vi "DIBPowerCheck_t.vi"(0 "TSM context":T2, 5 "DIBPowerCheck_TC":T1={"Voltage Limit, V"=24.0, "Current Level (A)"=0.05}) -> (15 "error out":errorcluster)   [LabVIEW 2019]
uses:
  <vilib>/NI_TestStand_SemiconductorModule/NI_TestStand_Semiconductor_Module.lvlibp/PinMap/General/SemiconductorModuleContext.ctl
  typedefs/DIBPowerCheck_TC.ctl
  typedefs/DIBPowerCheck_PC.ctl
  Common/Instrument Control/DCPower/TSM/TSM SSC DCPower.ctl
  <vilib>/NI_TestStand_SemiconductorModule/NI_TestStand_Semiconductor_Module.lvlibp/PinMap/PinQueryContext/MultiplePinMultipleSessionQueryContext/MultiplePinMultipleSessionQueryContext.lvclass
  C:/Program Files/National Instruments/LabVIEW 2019/vi.lib/NI_TestStand_SemiconductorModule/NI_TestStand_Semiconductor_Module.lvlibp/PinMap/PinQueryContext/PinQueryContext.lvclass
  Common/Instrument Control/DCPower/SSC DCPower/SSC DCPower.ctl
  Common/Instrument Control/Shared SubVIs/TSM Pin Abstraction/TSM Pin Information.ctl
  Common/Instrument Control/Shared SubVIs/TSM Pin Abstraction/TSM Pin Type Identifier.ctl
  Common/Instrument Control/Shared SubVIs/TSM Pin Abstraction/TSM Expanded Pin Information.ctl
  <instrlib>/niDCPower/nidcpower.llb/niDCPower Sense.ctl
  Common/Instrument Control/DCPower/SSC DCPower/Measure/SSC DCPower Measurement Mode.ctl
  <vilib>/Utility/High Resolution Polling Wait.vi
  Common/Instrument Control/DCPower/SSC DCPower/Control/SSC DCPower Abort.vi
  Common/Instrument Control/DCPower/SSC DCPower/Source/SSC DCPower Configure Output Connected.vi
  Common/Instrument Control/DCPower/SSC DCPower/Source/SSC DCPower Configure Output Enabled.vi
  <vilib>/NI_TestStand_SemiconductorModule/NI_TestStand_Semiconductor_Module.lvlibp/PinMap/General/Publish/PublishDataDouble1D.vi
  <vilib>/NI_TestStand_SemiconductorModule/NI_TestStand_Semiconductor_Module.lvlibp
  C:/Program Files/National Instruments/LabVIEW 2019/vi.lib/NI_TestStand_SemiconductorModule/NI_TestStand_Semiconductor_Module.lvlibp/PinMap/PinQueryContext/MultipleSessionPinQueryContext.lvclass
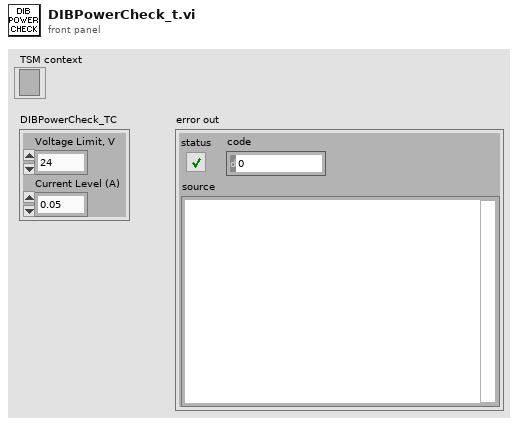
[diagram p1: front panel]
types:
  T1 = typedef "DIBPowerCheck_TC.ctl" = cluster{"Voltage Limit, V":dbl, "Current Level (A)":dbl}
  T2 = typedef "NI_TestStand_Semiconductor_Module.lvlibp/SemiconductorModuleContext.ctl" = refnum<k7>
  T3 = typedef "DIBPowerCheck_PC.ctl" = cluster{"DIB Supply Monitor":T4, "Site Numbers":i32[]}
  T4 = typedef "TSM SSC DCPower.ctl" = cluster{"Pin Query Context":refnum<class "MultiplePinMultipleSessionQueryContext.lvclass">, "SSC":T5[], "Site Numbers":i32[], "Pins":T6[], "Pins Expanded":T8[]}
  T5 = typedef "SSC DCPower.ctl" = cluster{"Session":refnum<k15>, "Chan":string, "Channel List":string}
  T6 = typedef "TSM Pin Information.ctl" = cluster{"Pin":tag, "Type":T7, "Count":i32}
  T7 = typedef "TSM Pin Type Identifier.ctl" = enum8{"DUT Pin", "System Pin", "Pin Group", "Not Determined"}
  T8 = typedef "TSM Expanded Pin Information.ctl" = cluster{"Pin":tag, "Type":T7, "Index":i32}
  T9 = cluster{"Measured Supply Voltages":dbl[], "DIBPowerCheck_TC":T1}
  T10 = typedef "SSC DCPower Measurement Mode.ctl" = enum16{"Auto", "Measure Multiple", "Software Triggers"}
  T11 = typedef "niDCPower Sense.ctl" = i32
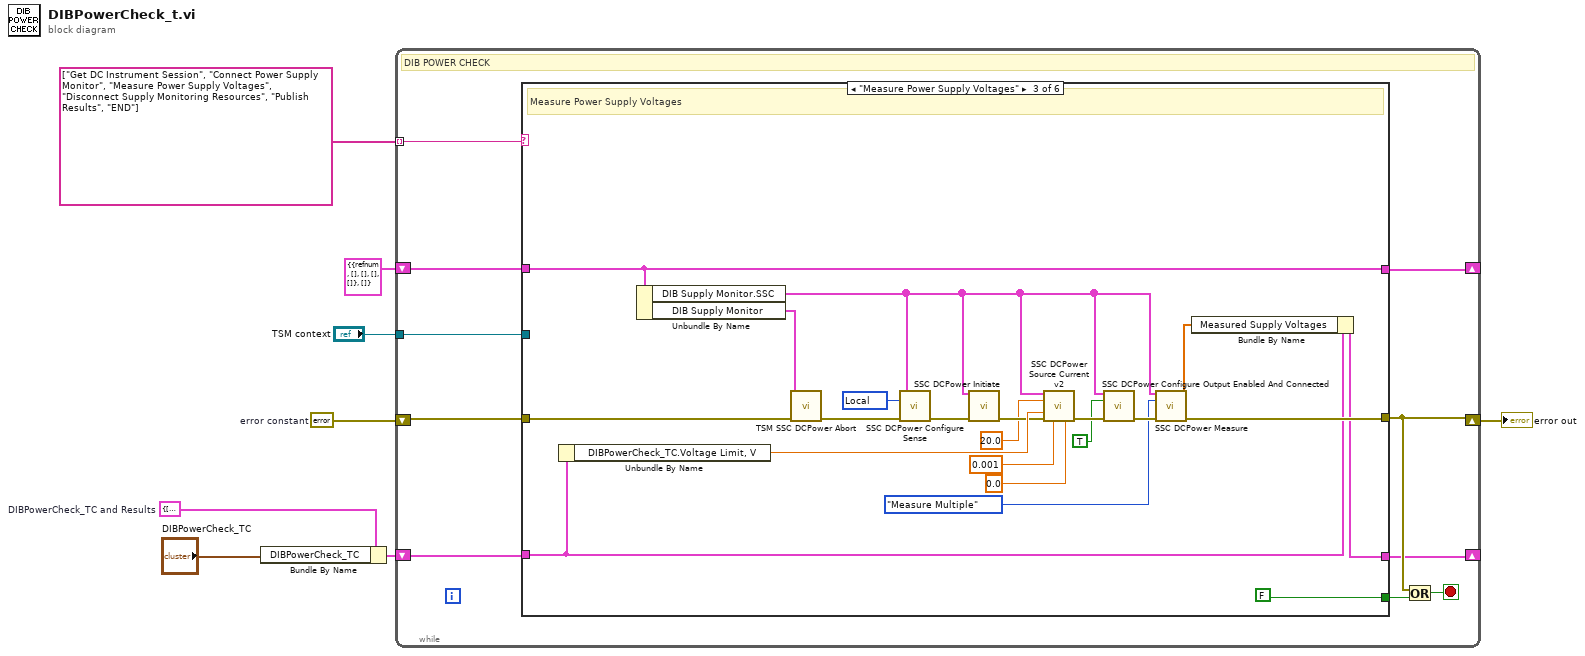
[diagram p0: block diagram]
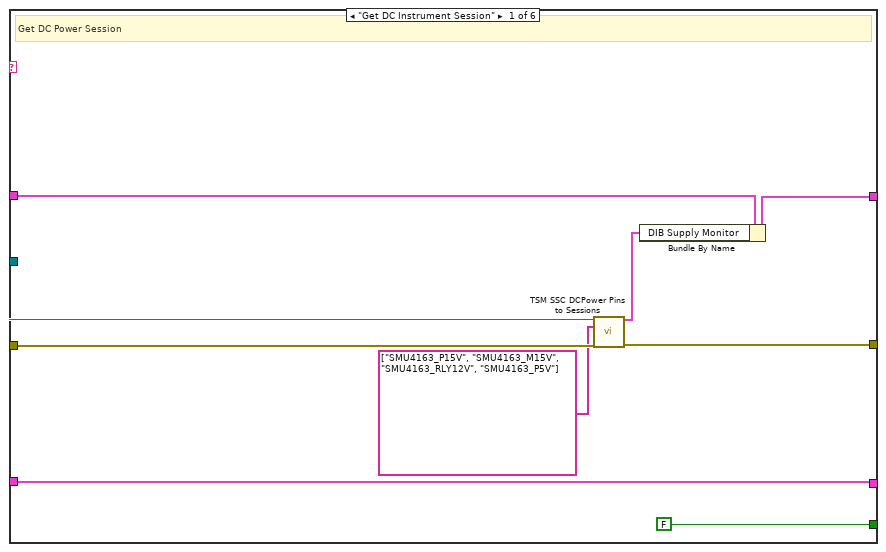
[diagram p2: hidden frame]
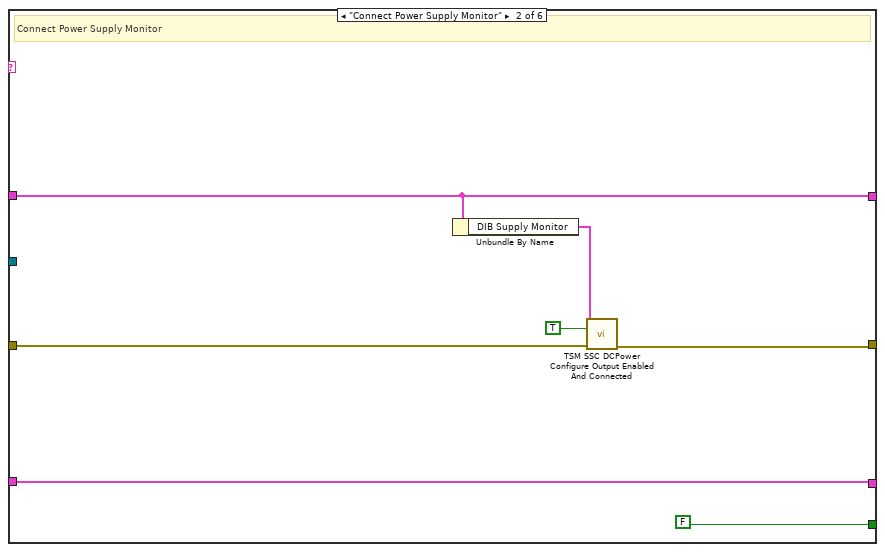
[diagram p3: hidden frame]
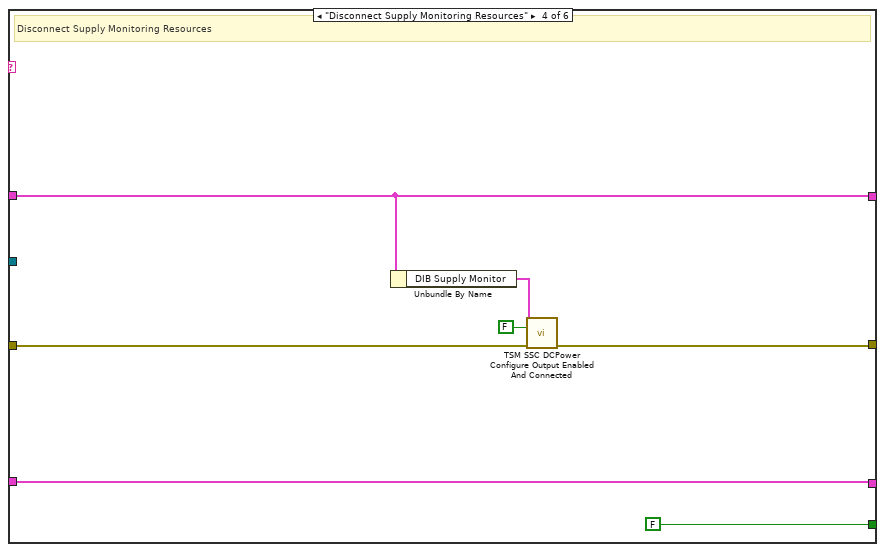
[diagram p4: hidden frame]
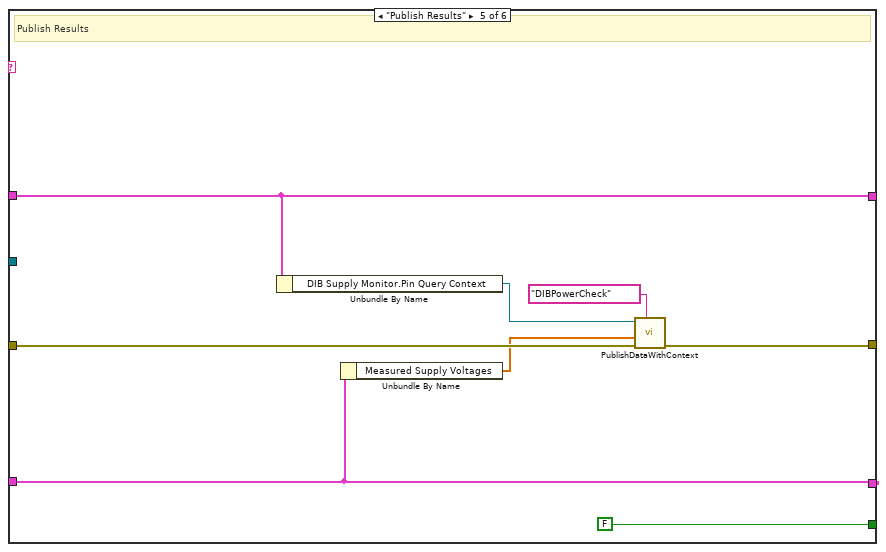
[diagram p5: hidden frame]
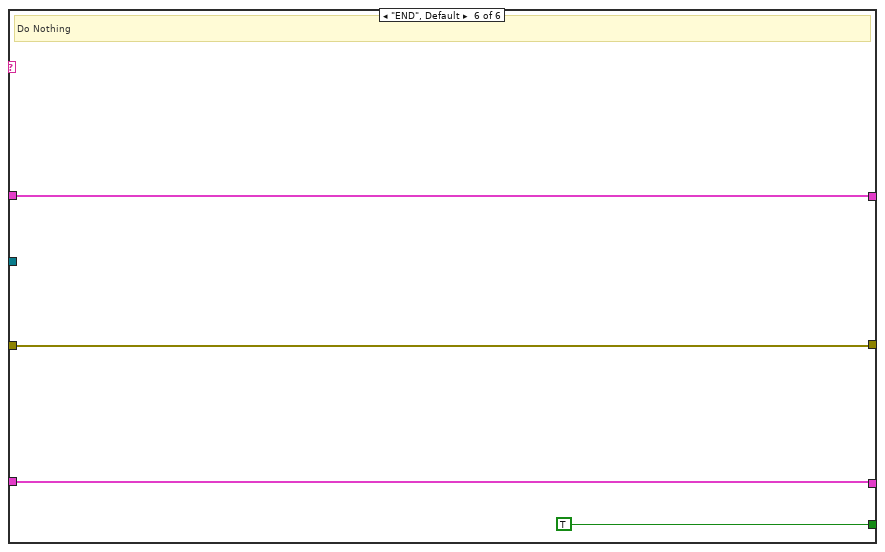
[diagram p6: hidden frame]
diagram:
  w7 = T9 {"Measured Supply Voltages"=[], "DIBPowerCheck_TC"={"Voltage Limit, V"=24.0, "Current Level (A)"=0.05}}  # DIBPowerCheck_TC and Results
  w4 = errorcluster {"status"=FALSE, "code"=0, "source"=""}  # error constant
  n1 = Bundle By Name(cluster=w7, "DIBPowerCheck_TC"="DIBPowerCheck_TC") -> (w6:T9)
  n2 = while {
    shift-right: [w14] -> w8
    shift-left: w4 -> [w18]
    tunnel: "TSM context" -> [w17]
    shift-right: [w15] -> _
    shift-left: T3 {"DIB Supply Monitor"={"Pin Query Context"=refnum, "SSC"=[], "Site Numbers"=[], "Pins"=[], "Pins Expanded"=[]}, "Site Numbers"=[]} ("Cluster") -> [w16]
    shift-right: [w10] -> _
    shift-left: w6 -> [w11]
    tunnel: string[] ["Get DC Instrument Session", "Connect Power Supply Monitor", "Measure Power Supply Voltages", "Disconnect Supply Monitoring Resources", "Publish Results", "END"] ("Test Flow") -> [w9] mode=indexing
    stop <- w12 stop-if-true
    # "DIB POWER CHECK"
    n3 = case shown="\"Measure Power Supply Voltages\"" w9 {
      tunnel: [FALSE FALSE FALSE FALSE FALSE TRUE] -> w13
      tunnel: w18 -> [w24 w34 w53 w62 w69 w73]
      tunnel: w17 -> [w20 _ _ _ _ _]
      tunnel: [w26 w30 w52 w61 w68 w73] -> w14
      tunnel: w16 -> [w23 w31 w55 w60 w66 w74]
      tunnel: [w22 w31 w55 w60 w66 w74] -> w15
      tunnel: w11 -> [w21 w33 w49 w57 w67 w72]
      tunnel: [w21 w33 w50 w57 w67 w72] -> w10
      frame "Get DC Instrument Session" {
        # "Get DC Power Session"
        n4 = call "TSM SSC DCPower Pins to Sessions.vi"("TSM context"=w20, "Pins"=tag[] ["SMU4163_P15V", "SMU4163_M15V", "SMU4163_RLY12V", "SMU4163_P5V"], "error in"=w24) -> ("DCPower TSM Out"=w25:T4, "error out"=w26:errorcluster)  [unwired: 11 in]
        n5 = Bundle By Name(cluster=w23, "DIB Supply Monitor"=w25) -> (w22:T3)
      }
      frame "Connect Power Supply Monitor" {
        # "Connect Power Supply Monitor"
        n6 = Unbundle By Name(w31) -> ("DIB Supply Monitor"=w29:T4)
        n7 = call "TSM SSC DCPower Configure Output Enabled And Connected.vi"("DCPower TSM in"=w29, "Output Enabled And Connected"=TRUE, "error in"=w34) -> ("error out"=w30:errorcluster)  [unwired: 11 in, 1 out]
      }
      frame "Measure Power Supply Voltages" {
        w44 = T11 1008 items=["Local"=1008, "Remote"=1009] ("Sense")
        # "Measure Power Supply Voltages"
        n8 = Unbundle By Name(w49) -> ("DIBPowerCheck_TC.Voltage Limit, V"=w48:dbl)
        n9 = Unbundle By Name(w55) -> ("DIB Supply Monitor.SSC"=w35:T5[], "DIB Supply Monitor"=w47:T4)
        n10 = call "TSM SSC DCPower Abort.vi"("DCPower TSM in"=w47, "error in"=w53) -> ("error out"=w46:errorcluster)  [unwired: 12 in, 1 out]
        n11 = call "SSC DCPower Configure Sense.vi"("DCPower SSC in"=w35, "Sense"=w44, "error in"=w46) -> ("error out"=w45:errorcluster)  [unwired: 11 in, 1 out]
        n12 = call "SSC DCPower Initiate.vi"("DCPower SSC in"=w35, "error in"=w45) -> ("error out"=w43:errorcluster)  [unwired: 12 in, 1 out]
        n13 = call "SSC DCPower Source Current v2.vi"("DCPower SSC in"=w35, "Voltage Limit, V"=20.0 ("Voltage Limit Range (V)"), "Voltage Limit Range (V)"=w48, "error in"=w43, "Current Level Range (A)"=0.001, "Current Level (A)"=0.0) -> ("error out"=w42:errorcluster)  [unwired: 8 in, 1 out]
        n14 = call "SSC DCPower Configure Output Enabled And Connected.vi"("DCPower SSC in"=w35, "Output Enabled And Connected"=TRUE, "error in"=w42) -> ("error out"=w41:errorcluster)  [unwired: 11 in, 1 out]
        n15 = call "SSC DCPower Measure.vi"("DCPower SSC in"=w35, "Measurement Mode"=SSC_DCPower_Measurement_Mode."Measure Multiple", "error in"=w41) -> ("Voltage Measurements (V)"=w51:dbl[], "error out"=w52:errorcluster)  [unwired: 9 in, 2 out]
        n16 = Bundle By Name(cluster=w49, "Measured Supply Voltages"=w51) -> (w50:T9)
      }
      frame "Disconnect Supply Monitoring Resources" {
        # "Disconnect Supply Monitoring Resources"
        n17 = Unbundle By Name(w60) -> ("DIB Supply Monitor"=w59:T4)
        n18 = call "TSM SSC DCPower Configure Output Enabled And Connected.vi"("DCPower TSM in"=w59, "Output Enabled And Connected"=FALSE, "error in"=w62) -> ("error out"=w61:errorcluster)  [unwired: 11 in, 1 out]
      }
      frame "Publish Results" {
        # "Publish Results"
        n19 = Unbundle By Name(w66) -> ("DIB Supply Monitor.Pin Query Context"=w64:refnum<class "MultiplePinMultipleSessionQueryContext.lvclass">)
        n20 = Unbundle By Name(w67) -> ("Measured Supply Voltages"=w65:dbl[])
        n21 = call-poly <vilib>:"PublishDataWithContext.vi"("Published Data Id"=tag "DIBPowerCheck", "error in (no error)"=w69, "Data In"=w65, "Pin Query Context"=w64) -> ("error out"=w68:errorcluster)  [unwired: 6 in, 1 out]
      }
      frame "END", Default {
        # "Do Nothing"
      }
    }
    n22 = Or(x=w14, y=w13) -> (x .or. y?=w12:bool)
  }
  "error out" <- w8
